vi "Update Data.vi"(8 "error in (no error)":errorcluster, 10 "Generic Data Type":refnum<class "Generic Data Type.lvclass">, 11 "DataGrid Config Dialog in":refnum<class "DataGrid Config Dialog.lvclass">) -> (0 "error out":errorcluster, 3 "DataGrid Config Dialog out":refnum<class "DataGrid Config Dialog.lvclass">)   [LabVIEW 2018, in "DataGrid Config Dialog.lvclass"]
uses:
  DataGrid Config Dialog.lvclass
  Data Type Classes/Generic/Generic Data Type.lvclass
  DataGrid Config Dialog.lvclass/DataGrid Config Dialog.ctl
  DataGrid Config/Edit Configuration Actions.ctl
  DataGrid Config/DataGrid Config.lvclass
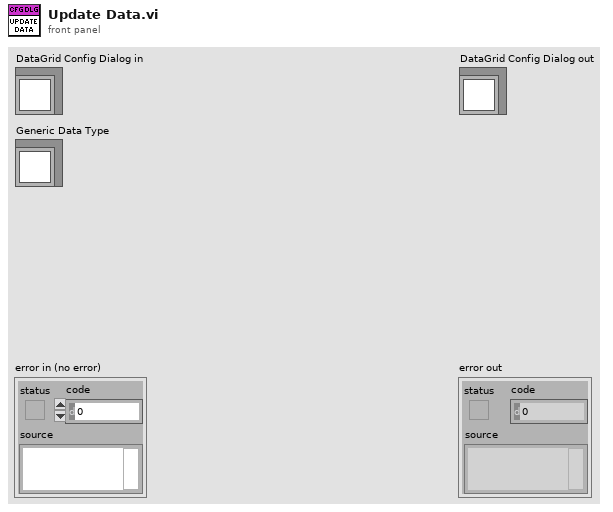
[diagram p1: front panel]
types:
  T1 = typedef "DataGrid Config.lvclass/Edit Configuration Actions.ctl" = enum16{"Add", "Remove", "Update", "Move Up", "Move Down"}
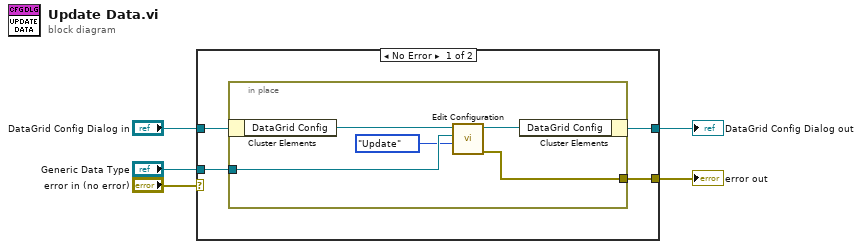
[diagram p0: block diagram]
diagram:
  n1 = case shown="No Error" "error in (no error)" {
    selector: "error in (no error)" -> [_ w16]
    tunnel: [w6 w16] -> w4
    tunnel: [w8 w15] -> w2
    tunnel: "DataGrid Config Dialog in" -> [w9 w15]
    tunnel: "Generic Data Type" -> [w7 _]
    frame No Error {
      n2 = in-place {
        in-place-border: w7 -> [w11]
        in-place-border: [w12] -> w6
        n3 = in-place-cluster #1(w9) -> ("DataGrid Config"=w14:refnum<class "DataGrid Config.lvclass">)
        n4 = call "Edit Configuration.vi"("Edit Configuration Actions"=Edit_Configuration_Actions."Update", "Data Type Object"=w11, "DataGrid Config in"=w14) -> ("error out"=w12:errorcluster, "DataGrid Config out"=w13:refnum<class "DataGrid Config.lvclass">)  [unwired: 7 in]
        n5 = in-place-cluster #1("DataGrid Config"=w13) -> (w8:refnum<class "DataGrid Config Dialog.lvclass">)
      }
    }
    frame Error {
    }
  }
  "error out" <- w4
  "DataGrid Config Dialog out" <- w2
